vi "2_valve_control.vi"() -> ()   [LabVIEW 2014]
uses:
  <vilib>/DAQmx/write.llb/DAQmx Write (Digital Bool 1Line 1Point).vi
panel:
  out "State:":T1(ring)
  in  "Continuous\ngeneration":bool
  in  "Waiting time 2":dbl
  in  "Waiting time 1":dbl
  out "Valve 2":bool
  out "Valve1":bool
  in  "Time L2":dbl
  in  "Time L1":dbl
  in  "Repetitions":dbl
  in  "stop":bool
  in  "Limited\ngeneration":bool
  in  "Valve 2":bool
  in  "Valve 1":bool
  # "Automatic Generator - set parameters:"
  # "Manual Control"
  # "ms"
  # "ms"
  # "ms"
  # "ms"
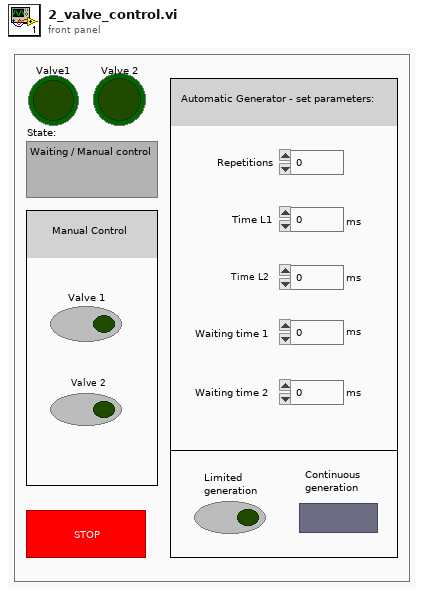
[diagram p1: front panel]
types:
  T1 = enum16{"Waiting / Manual control", "Limited generation", "Continuous Generation"}
  T2 = cluster{"Valve 1":bool, "Valve 2":bool, "stop":bool}
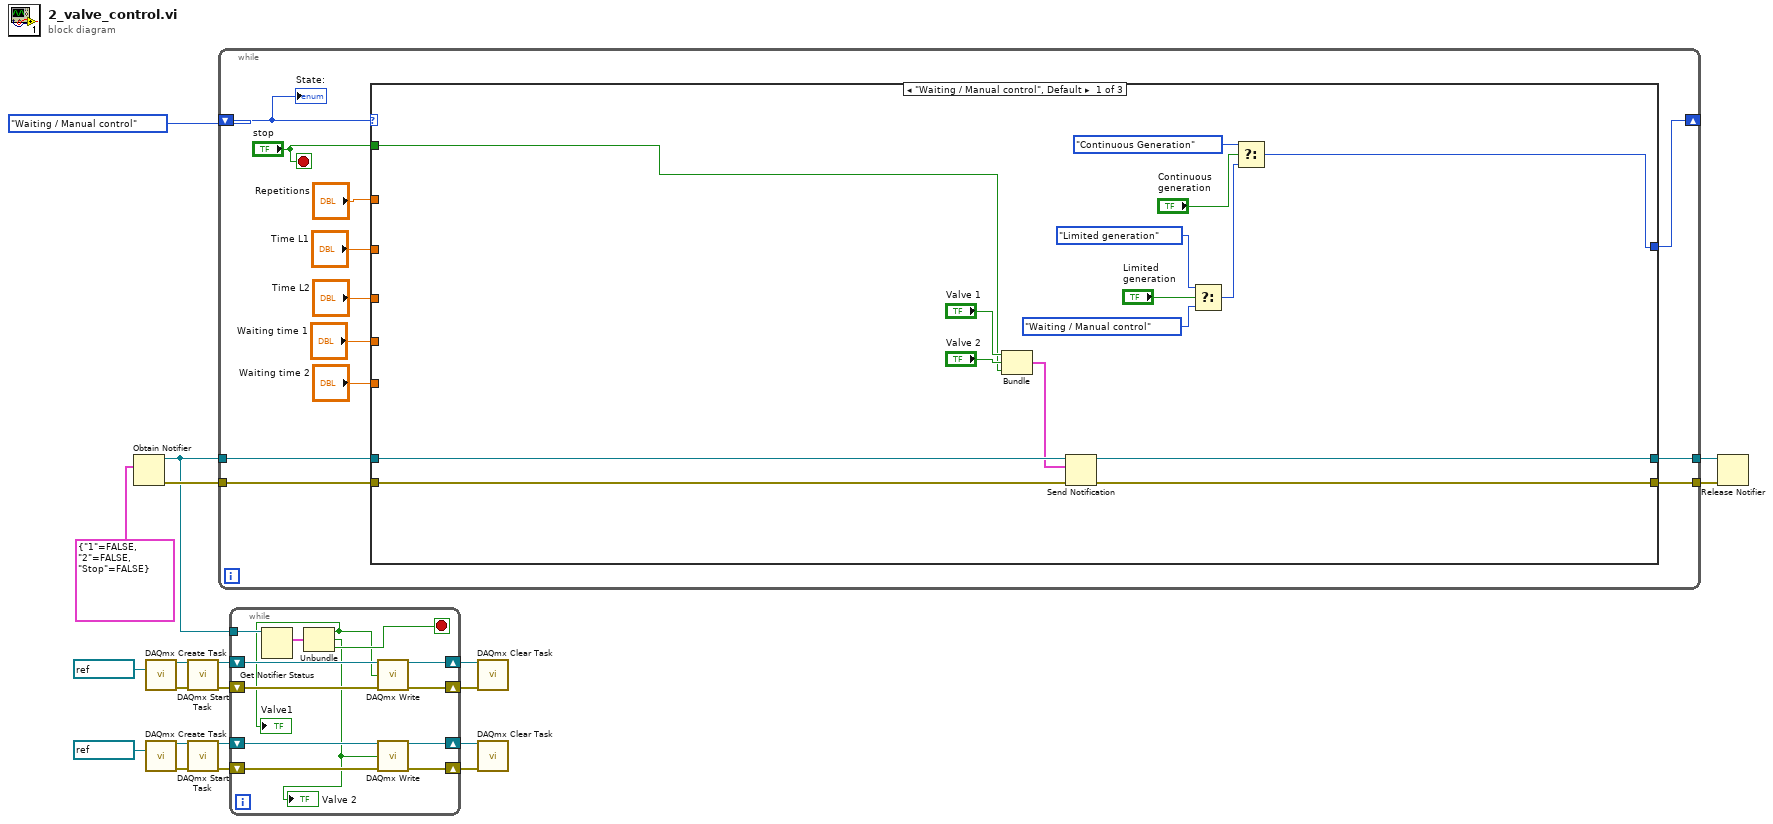
[diagram p0: block diagram]
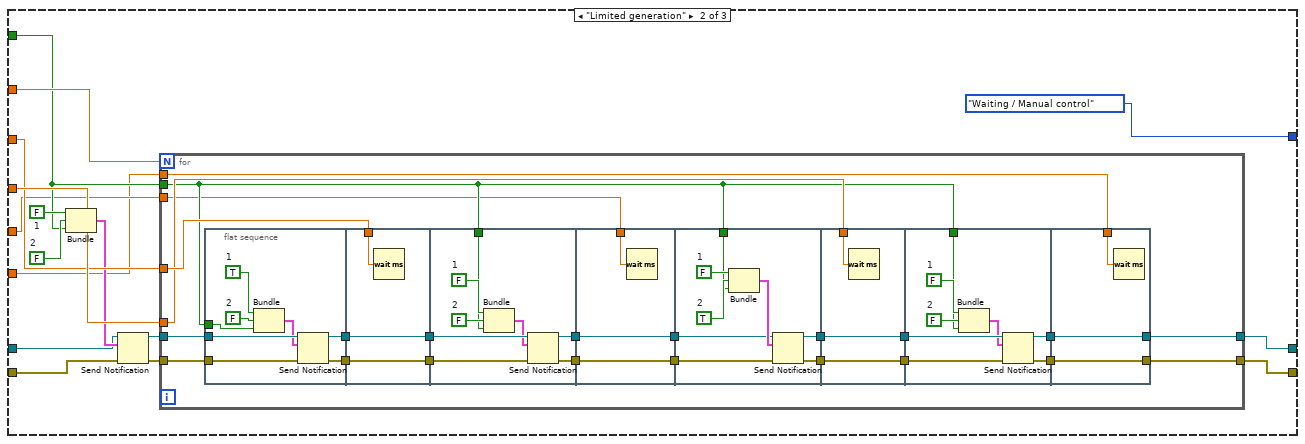
[diagram p2: hidden frame]
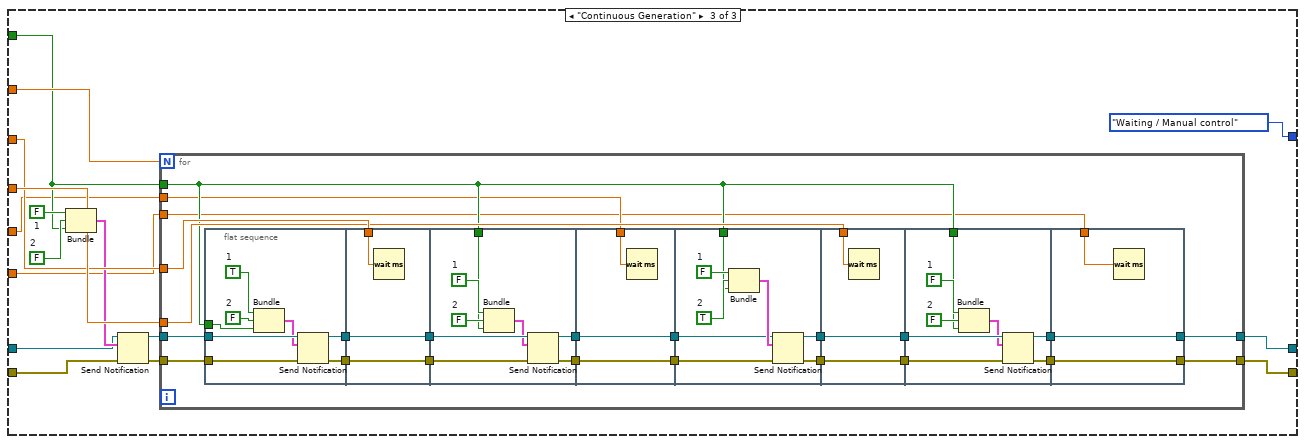
[diagram p3: hidden frame]
diagram:
  n1 = Obtain Notifier(notification data type=cluster{"1":bool, "2":bool, "Stop":bool} {"1"=FALSE, "2"=FALSE, "Stop"=FALSE}) -> (notifier out=w1:refnum<notifier>, error out=w4:errorcluster)  [unwired: 3 in, 1 out]
  n2 = call <vilib>:"DAQmx Create Task.vi"("task to copy"=refnum<k21> "valve1") -> ("task out"=w14:refnum<k21>, "error out"=w15:errorcluster)  [unwired: 13 in]
  n3 = call <vilib>:"DAQmx Create Task.vi"("task to copy"=refnum<k21> "valve2") -> ("task out"=w19:refnum<k21>, "error out"=w18:errorcluster)  [unwired: 13 in]
  n4 = call <vilib>:"DAQmx Start Task.vi"("task/channels in"=w14, "error in"=w15) -> ("task out"=w13:refnum<k21>, "error out"=w12:errorcluster)  [unwired: 12 in]
  n5 = call <vilib>:"DAQmx Start Task.vi"("task/channels in"=w19, "error in"=w18) -> ("task out"=w11:refnum<k21>, "error out"=w10:errorcluster)  [unwired: 12 in]
  n6 = while {
    shift-right: [w32] -> _
    shift-left: T1."Waiting / Manual control" ("State:") -> [w21]
    tunnel: w1 -> [w31]
    tunnel: w4 -> [w30]
    tunnel: [w28] -> w3
    tunnel: [w29] -> w2
    stop <- "stop" stop-if-true
    n7 = case shown="\"Waiting / Manual control\", Default" w21 {
      tunnel: [w33 T1."Waiting / Manual control" ("State:") T1."Waiting / Manual control" ("State:")] -> w32
      tunnel: w31 -> [w45 w56 w139]
      tunnel: w30 -> [w44 w57 w140]
      tunnel: [w42 w53 w136] -> w28
      tunnel: [w41 w52 w135] -> w29
      tunnel: "stop" -> [w40 w51 w134]
      tunnel: "Repetitions" -> [_ w63 w146]
      tunnel: "Time L2" -> [_ w62 w145]
      tunnel: "Time L1" -> [_ w61 w144]
      tunnel: "Waiting time 1" -> [_ w49 w132]
      tunnel: "Waiting time 2" -> [_ w48 w131]
      frame "Waiting / Manual control", Default {
        n8 = Bundle("Valve 1"="Valve 1", "Valve 2"="Valve 2", "stop"=w40) -> (w43:T2)  [unwired: 1 in]
        n9 = Send Notification(notification=w43, notifier=w45, error in (no error)=w44) -> (notifier out=w42:refnum<notifier>, error out=w41:errorcluster)
        n10 = Select(t=T1."Limited generation" ("State:"), s="Limited\ngeneration", f=T1."Waiting / Manual control" ("State:")) -> (s? t:f=w36:T1)
        n11 = Select(t=T1."Continuous Generation" ("State:"), s="Continuous\ngeneration", f=w36) -> (s? t:f=w33:T1)
      }
      frame "Limited generation" {
        w59 = FALSE  # 2
        w60 = FALSE  # 1
        n12 = Bundle("1"=w60, "2"=w59, "stop"=w51) -> (w58:cluster{"1":bool, "2":bool, "stop":bool})  [unwired: 1 in]
        n13 = Send Notification(notification=w58, notifier=w56, error in (no error)=w57) -> (notifier out=w55:refnum<notifier>, error out=w54:errorcluster)
        n14 = for {
          N: w63 -> [_]
          tunnel: w55 -> [w67]
          tunnel: w54 -> [w66]
          tunnel: w51 -> [w68]
          tunnel: w61 -> [w82]
          tunnel: w62 -> [w81]
          tunnel: [w70] -> w52
          tunnel: [w69] -> w53
          tunnel: w49 -> [w65]
          tunnel: w48 -> [w64]
          n15 = flat-sequence {
            tunnel: w68 -> [w87]
            tunnel: w67 -> [w92]
            tunnel: w66 -> [w91]
            tunnel: [w89] -> w86
            tunnel: [w88] -> w85
            tunnel: [w97] -> w80
            tunnel: w86 -> [w97]
            tunnel: [w96] -> w79
            tunnel: w85 -> [w96]
            tunnel: w82 -> [w95]
            tunnel: w80 -> [w105]
            tunnel: w79 -> [w104]
            tunnel: [w103] -> w78
            tunnel: [w102] -> w76
            tunnel: w68 -> [w98]
            tunnel: w78 -> [w108]
            tunnel: [w108] -> w77
            tunnel: w76 -> [w107]
            tunnel: [w107] -> w75
            tunnel: w65 -> [w106]
            tunnel: w68 -> [w109]
            tunnel: [w111] -> w84
            tunnel: [w110] -> w83
            tunnel: w77 -> [w113]
            tunnel: w75 -> [w112]
            tunnel: w84 -> [w119]
            tunnel: w83 -> [w118]
            tunnel: w81 -> [w117]
            tunnel: [w119] -> w74
            tunnel: [w118] -> w73
            tunnel: w74 -> [w124]
            tunnel: w73 -> [w125]
            tunnel: w68 -> [w120]
            tunnel: [w122] -> w72
            tunnel: [w121] -> w71
            tunnel: w72 -> [w129]
            tunnel: w71 -> [w130]
            tunnel: [w130] -> w70
            tunnel: [w129] -> w69
            tunnel: w64 -> [w128]
            frame #0 {
              w93 = FALSE  # 2
              w94 = TRUE  # 1
              n16 = Bundle("1"=w94, "2"=w93, "stop"=w87) -> (w90:cluster{"1":bool, "2":bool, "stop":bool})  [unwired: 1 in]
              n17 = Send Notification(notification=w90, notifier=w92, error in (no error)=w91) -> (notifier out=w89:refnum<notifier>, error out=w88:errorcluster)
            }
            frame #1 {
              n18 = Wait (ms)(milliseconds to wait=w95) -> ()  [unwired: 1 out]
            }
            frame #2 {
              w100 = FALSE  # 2
              w101 = FALSE  # 1
              n19 = Bundle("1"=w101, "2"=w100, "stop"=w98) -> (w99:cluster{"1":bool, "2":bool, "stop":bool})  [unwired: 1 in]
              n20 = Send Notification(notification=w99, notifier=w105, error in (no error)=w104) -> (notifier out=w103:refnum<notifier>, error out=w102:errorcluster)
            }
            frame #3 {
              n21 = Wait (ms)(milliseconds to wait=w106) -> ()  [unwired: 1 out]
            }
            frame #4 {
              w115 = TRUE  # 2
              w116 = FALSE  # 1
              n22 = Bundle("1"=w116, "2"=w115, "stop"=w109) -> (w114:cluster{"1":bool, "2":bool, "stop":bool})  [unwired: 1 in]
              n23 = Send Notification(notification=w114, notifier=w113, error in (no error)=w112) -> (notifier out=w110:refnum<notifier>, error out=w111:errorcluster)
            }
            frame #5 {
              n24 = Wait (ms)(milliseconds to wait=w117) -> ()  [unwired: 1 out]
            }
            frame #6 {
              w127 = FALSE  # 2
              w126 = FALSE  # 1
              n25 = Bundle("1"=w126, "2"=w127, "stop"=w120) -> (w123:cluster{"1":bool, "2":bool, "stop":bool})  [unwired: 1 in]
              n26 = Send Notification(notification=w123, notifier=w125, error in (no error)=w124) -> (notifier out=w122:refnum<notifier>, error out=w121:errorcluster)
            }
            frame #7 {
              n27 = Wait (ms)(milliseconds to wait=w128) -> ()  [unwired: 1 out]
            }
          }
        }
      }
      frame "Continuous Generation" {
        w142 = FALSE  # 2
        w143 = FALSE  # 1
        n28 = Bundle("1"=w143, "2"=w142, "stop"=w134) -> (w141:cluster{"1":bool, "2":bool, "stop":bool})  [unwired: 1 in]
        n29 = Send Notification(notification=w141, notifier=w139, error in (no error)=w140) -> (notifier out=w138:refnum<notifier>, error out=w137:errorcluster)
        n30 = for {
          N: w146 -> [_]
          tunnel: w138 -> [w150]
          tunnel: w137 -> [w149]
          tunnel: w134 -> [w151]
          tunnel: w144 -> [w165]
          tunnel: w145 -> [w164]
          tunnel: [w153] -> w135
          tunnel: [w152] -> w136
          tunnel: w132 -> [w148]
          tunnel: w131 -> [w147]
          n31 = flat-sequence {
            tunnel: w151 -> [w170]
            tunnel: w150 -> [w175]
            tunnel: w149 -> [w174]
            tunnel: [w172] -> w169
            tunnel: [w171] -> w168
            tunnel: [w180] -> w163
            tunnel: w169 -> [w180]
            tunnel: [w179] -> w162
            tunnel: w168 -> [w179]
            tunnel: w165 -> [w178]
            tunnel: w163 -> [w188]
            tunnel: w162 -> [w187]
            tunnel: [w186] -> w161
            tunnel: [w185] -> w159
            tunnel: w151 -> [w181]
            tunnel: w161 -> [w191]
            tunnel: [w191] -> w160
            tunnel: w159 -> [w190]
            tunnel: [w190] -> w158
            tunnel: w148 -> [w189]
            tunnel: w151 -> [w192]
            tunnel: [w194] -> w167
            tunnel: [w193] -> w166
            tunnel: w160 -> [w196]
            tunnel: w158 -> [w195]
            tunnel: w167 -> [w202]
            tunnel: w166 -> [w201]
            tunnel: w164 -> [w200]
            tunnel: [w202] -> w157
            tunnel: [w201] -> w156
            tunnel: w157 -> [w207]
            tunnel: w156 -> [w208]
            tunnel: w151 -> [w203]
            tunnel: [w205] -> w155
            tunnel: [w204] -> w154
            tunnel: w155 -> [w212]
            tunnel: w154 -> [w213]
            tunnel: [w213] -> w153
            tunnel: [w212] -> w152
            tunnel: w147 -> [w211]
            frame #0 {
              w176 = FALSE  # 2
              w177 = TRUE  # 1
              n32 = Bundle("1"=w177, "2"=w176, "stop"=w170) -> (w173:cluster{"1":bool, "2":bool, "stop":bool})  [unwired: 1 in]
              n33 = Send Notification(notification=w173, notifier=w175, error in (no error)=w174) -> (notifier out=w172:refnum<notifier>, error out=w171:errorcluster)
            }
            frame #1 {
              n34 = Wait (ms)(milliseconds to wait=w178) -> ()  [unwired: 1 out]
            }
            frame #2 {
              w183 = FALSE  # 2
              w184 = FALSE  # 1
              n35 = Bundle("1"=w184, "2"=w183, "stop"=w181) -> (w182:cluster{"1":bool, "2":bool, "stop":bool})  [unwired: 1 in]
              n36 = Send Notification(notification=w182, notifier=w188, error in (no error)=w187) -> (notifier out=w186:refnum<notifier>, error out=w185:errorcluster)
            }
            frame #3 {
              n37 = Wait (ms)(milliseconds to wait=w189) -> ()  [unwired: 1 out]
            }
            frame #4 {
              w198 = TRUE  # 2
              w199 = FALSE  # 1
              n38 = Bundle("1"=w199, "2"=w198, "stop"=w192) -> (w197:cluster{"1":bool, "2":bool, "stop":bool})  [unwired: 1 in]
              n39 = Send Notification(notification=w197, notifier=w196, error in (no error)=w195) -> (notifier out=w193:refnum<notifier>, error out=w194:errorcluster)
            }
            frame #5 {
              n40 = Wait (ms)(milliseconds to wait=w200) -> ()  [unwired: 1 out]
            }
            frame #6 {
              w210 = FALSE  # 2
              w209 = FALSE  # 1
              n41 = Bundle("1"=w209, "2"=w210, "stop"=w203) -> (w206:cluster{"1":bool, "2":bool, "stop":bool})  [unwired: 1 in]
              n42 = Send Notification(notification=w206, notifier=w208, error in (no error)=w207) -> (notifier out=w205:refnum<notifier>, error out=w204:errorcluster)
            }
            frame #7 {
              n43 = Wait (ms)(milliseconds to wait=w211) -> ()  [unwired: 1 out]
            }
          }
        }
      }
    }
    "State:" <- w21
  }
  n44 = while {
    shift-right: [w220] -> w6
    shift-left: w10 -> [w223]
    shift-right: [w221] -> w7
    shift-left: w11 -> [w224]
    shift-right: [w219] -> w8
    shift-left: w12 -> [w225]
    shift-right: [w222] -> w9
    shift-left: w13 -> [w226]
    tunnel: w1 -> [w218]
    stop <- w216 stop-if-true
    n45 = Get Notifier Status(notifier=w218) -> (current notification=w217:cluster{"1":bool, "2":bool, "Stop":bool})  [unwired: 1 in, 4 out]
    n46 = Unbundle(w217) -> ("1"=w215:bool, "2"=w214:bool, "Stop"=w216:bool)
    "Valve1" <- w215
    "Valve 2" <- w214
    n47 = call-poly <vilib>:"DAQmx Write.vi"("task/channels in"=w226, "data"=w215, "error in"=w225) -> ("task out"=w222:refnum<k21>, "error out"=w219:errorcluster)  [unwired: 10 in, 1 out]
    n48 = call-poly <vilib>:"DAQmx Write.vi"("task/channels in"=w224, "data"=w214, "error in"=w223) -> ("task out"=w221:refnum<k21>, "error out"=w220:errorcluster)  [unwired: 10 in, 1 out]
  }
  n49 = call <vilib>:"DAQmx Clear Task.vi"("task in"=w9, "error in"=w8) -> ()  [unwired: 13 in, 1 out]
  n50 = call <vilib>:"DAQmx Clear Task.vi"("task in"=w7, "error in"=w6) -> ()  [unwired: 13 in, 1 out]
  n51 = Release Notifier(notifier=w3, error in (no error)=w2) -> ()  [unwired: 1 in, 3 out]
